vi "collectFrame.vi"(7 "Reset":bool, 8 "error in (no error)":errorcluster, 10 "byte":u8, 11 "Modbus in":refnum<class "Modbus.lvclass">) -> (0 "error out":errorcluster, 1 "Data":i16[](array[numeric]), 2 "Finished":bool, 3 "Modbus out":refnum<class "Modbus.lvclass">, 5 "OK?":bool)   [LabVIEW 2015, in "ModBUS.lvlib" / "Modbus.lvclass"]
uses:
  Modbus.lvclass
panel:
  out "Function":u8
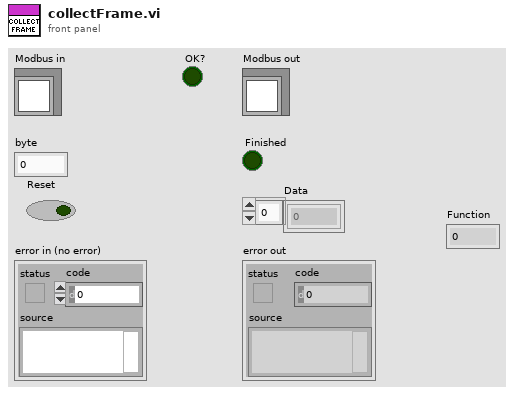
[diagram p1: front panel]
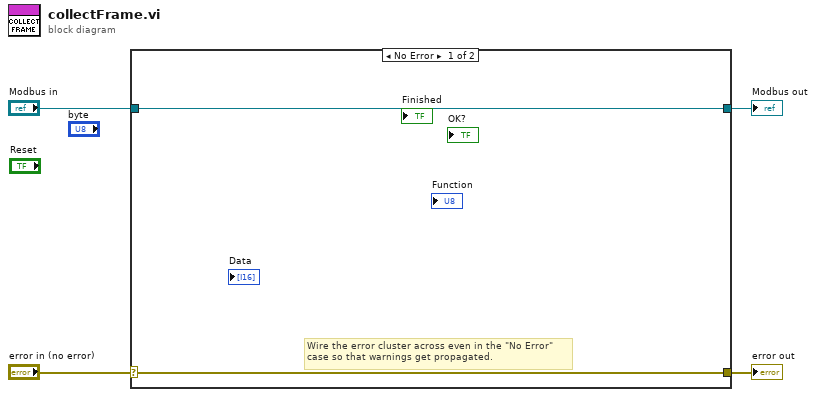
[diagram p0: block diagram]
diagram:
  n1 = case shown="No Error" "error in (no error)" {
    selector: "error in (no error)" -> [w5 w8]
    tunnel: [w5 w8] -> w3
    tunnel: [w6 w7] -> w1
    tunnel: "Modbus in" -> [w6 w7]
    frame No Error {
      # "Wire the error cluster across even in the \"No Error\"\ncase so that warnings get propagated."
    }
    frame Error {
    }
  }
  "error out" <- w3
  "Modbus out" <- w1
